vi "Shooting Shoot.vi"(10 "Power":dbl, 11 "error in (no error)":errorcluster) -> (3 "error out":errorcluster)   [LabVIEW 2015]
uses:
  References/Refnums.vi
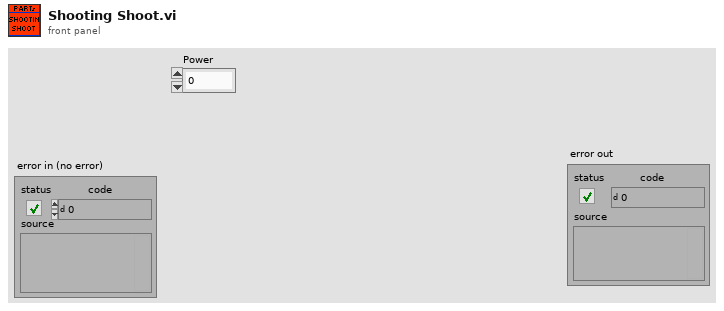
[diagram p1: front panel]
types:
  T1 = typedef "WPI_MotorControlDeviceRef.ctl" = cluster{"DeviceStatus":errorcluster, "Type":T2, "PWM":cluster{"PWM Channel":T3, "DeadBand":T4}, "CAN":cluster{"Device Number":u8, "Control Mode":T5, "Semaphore":T6, "Max Vout":dbl, "TalonSRX Control Mode":T7}, "Invert":bool}
  T2 = typedef "WPI_MotorControlType.ctl" = enum16{"PWM", "CAN", "CANTalonSRX"}
  T3 = typedef "FPGA_DIOPWMChannel.ctl" = enum8{"PWM 0", "PWM 1", "PWM 2", "PWM 3", "PWM 4", "PWM 5", "PWM 6", "PWM 7", "PWM 8", "PWM 9", "PWM MXP 0", "PWM MXP 1", "PWM MXP 2", "PWM MXP 3", "PWM MXP 4", "PWM MXP 5", "PWM MXP 6", "PWM MXP 7", "PWM MXP 8", "PWM MXP 9", "Invalid"}
  T4 = typedef "WPI_PWMDeadband.ctl" = cluster{"Name":string, "maxPositivePwm":i32, "minPositivePwm":i32, "centerPwm":i32, "maxNegativePwm":i32, "minNegativePwm":i32, "angularRange":u16}
  T5 = typedef "WPI_CANJaguar_ControlMode.ctl" = enum8{"Percent VBus", "Current", "Speed", "Position", "Voltage"}
  T6 = typedef "Semaphore RefNum" = refnum<k1>
  T7 = typedef "WPI_CANTalonSRX_APIControlMode.ctl" = enum8{"Percent VBus", "Speed", "Position", "Slave", "Unchanged / Invalid", "Voltage Compensation", "Current", "Motion Profile"}
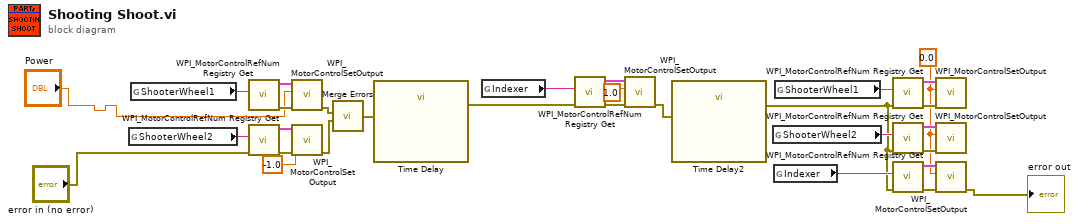
[diagram p0: block diagram]
diagram:
  w6 = 0.0
  n1 = global read "Refnums.vi" "ShooterWheel2"() -> (w28:string)
  n2 = global read "Refnums.vi" "ShooterWheel1"() -> (w27:string)
  n3 = call <vilib>:"WPI_MotorControlRefNum Registry Get.vi"("refnum name"=w27) -> ("error out"=w25:errorcluster, "MotorControlDevRef"=w26:T1)  [unwired: 9 in]
  n4 = call <vilib>:"WPI_MotorControlRefNum Registry Get.vi"("error in (no error)"="error in (no error)", "refnum name"=w28) -> ("error out"=w29:errorcluster, "MotorControlDevRef"=w30:T1)  [unwired: 8 in]
  n5 = call <vilib>:"WPI_MotorControlSetOutput.vi"("error in (no error)"=w25, "Output"="Power", "MotorControlDevRef"=w26) -> ("error out"=w24:errorcluster)  [unwired: 6 in, 2 out]
  n6 = call <vilib>:"WPI_MotorControlSetOutput.vi"("error in (no error)"=w29, "Output"=-1.0, "MotorControlDevRef"=w30) -> ("error out"=w23:errorcluster)  [unwired: 6 in, 2 out]
  n7 = call "Merge Errors.vi"("error in 2"=w23, "error in"=w24) -> ("error out"=w22:errorcluster)  [unwired: 2 in]
  n8 = call "Time Delay"("error in (no error)"=w22) -> ("error out"=w18:errorcluster)  [unwired: 10 in]
  n9 = global read "Refnums.vi" "Indexer"() -> (w19:string)
  n10 = call <vilib>:"WPI_MotorControlRefNum Registry Get.vi"("error in (no error)"=w18, "refnum name"=w19) -> ("error out"=w21:errorcluster, "MotorControlDevRef"=w20:T1)  [unwired: 8 in]
  n11 = call <vilib>:"WPI_MotorControlSetOutput.vi"("error in (no error)"=w21, "Output"=1.0, "MotorControlDevRef"=w20) -> ("error out"=w16:errorcluster)  [unwired: 6 in, 2 out]
  n12 = call "Time Delay2"("error in (no error)"=w16) -> ("error out"=w5:errorcluster)  [unwired: 10 in]
  n13 = global read "Refnums.vi" "ShooterWheel2"() -> (w13:string)
  n14 = global read "Refnums.vi" "Indexer"() -> (w7:string)
  n15 = global read "Refnums.vi" "ShooterWheel1"() -> (w12:string)
  n16 = call <vilib>:"WPI_MotorControlRefNum Registry Get.vi"("error in (no error)"=w5, "refnum name"=w12) -> ("error out"=w10:errorcluster, "MotorControlDevRef"=w11:T1)  [unwired: 8 in]
  n17 = call <vilib>:"WPI_MotorControlRefNum Registry Get.vi"("error in (no error)"=w5, "refnum name"=w13) -> ("error out"=w14:errorcluster, "MotorControlDevRef"=w15:T1)  [unwired: 8 in]
  n18 = call <vilib>:"WPI_MotorControlRefNum Registry Get.vi"("error in (no error)"=w5, "refnum name"=w7) -> ("error out"=w9:errorcluster, "MotorControlDevRef"=w8:T1)  [unwired: 8 in]
  n19 = call <vilib>:"WPI_MotorControlSetOutput.vi"("error in (no error)"=w10, "Output"=w6, "MotorControlDevRef"=w11) -> ()  [unwired: 6 in, 3 out]
  n20 = call <vilib>:"WPI_MotorControlSetOutput.vi"("error in (no error)"=w14, "Output"=w6, "MotorControlDevRef"=w15) -> ()  [unwired: 6 in, 3 out]
  n21 = call <vilib>:"WPI_MotorControlSetOutput.vi"("error in (no error)"=w9, "Output"=w6, "MotorControlDevRef"=w8) -> ("error out"=→"error out":errorcluster)  [unwired: 6 in, 2 out]
